vi "DAQ_ChannelReadBlock.vi"(0 "User Signal ID":i32, 1 "Count":i32, 2 "Time stamps":dbl[](array[numeric]), 3 "Values":dbl[](array[numeric])) -> (7 "Read block":T1)   [LabVIEW 2016]
uses:
  DAQ_ReadBlock.ctl
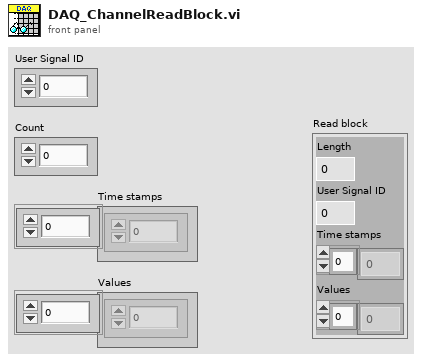
[diagram p1: front panel]
types:
  T1 = typedef "DAQ_ReadBlock.ctl" = cluster{"Length":i32, "User Signal ID":i32, "Time stamps":dbl[], "Values":dbl[]}
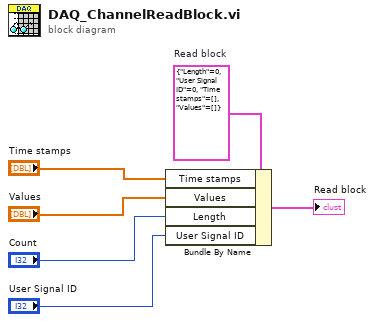
[diagram p0: block diagram]
diagram:
  w5 = T1 {"Length"=0, "User Signal ID"=0, "Time stamps"=[], "Values"=[]}  # Read block
  n1 = Bundle By Name(cluster=w5, "Time stamps"="Time stamps", "Values"="Values", "Length"="Count", "User Signal ID"="User Signal ID") -> (→"Read block":T1)
